vi "Set Color Table.vi"(10 "Color Table":T1={"Occupied Color"={"Value"=0, "Color"=0}, "Free Color"={"Value"=205, "Color"=16777215}, "Unknown Color"={"Value"=254, "Color"=13421772}}, 11 "Map Model in":refnum<class "Map Model.lvclass">) -> (3 "Map Model out":refnum<class "Map Model.lvclass">)   [LabVIEW 2020, in "Map Model.lvlib" / "Map Model.lvclass"]
uses:
  Map Model.lvclass
  Map Model.lvclass/Map Model.ctl
panel:
  # "NOTICE -- YOU MUST LEAVE THIS NOTICE IN PLACE.\n\nCopyright (c) 2017, LIANG LIU Shawn.Liu.cn@gmail.com\nAll rights reserved.\n\nRedistribution and use in source and binary forms, with or without modification, are permitted provided that the following conditions are met:\n-Redistributions of source code must retain the above copyright notice, this list of conditions and the following disclaimer.\n-Redistributions in binary form must reproduce the above copyright notice, this list of conditions and the following disclaimer in the documentation and/or other materials provided with the distribution.\n-Neither the name of the eLp nor the names of its contributors may be used to endorse or promote products derived from this software without specific prior written permission.\n\nTHIS SOFTWARE IS PROVIDED BY THE COPYRIGHT HOLDERS AND CONTRIBUTORS \"AS IS\" AND ANY EXPRESS OR IMPLIED WARRANTIES, INCLUDING, BUT NOT LIMITED TO, THE IMPLIED WARRANTIES OF MERCHANTABILITY AND FITNESS FOR A PARTICULAR PURPOSE ARE DISCLAIMED. IN NO EVENT SHALL THE COPYRIGHT HOLDER OR CONTRIBUTORS BE LIABLE FOR ANY DIRECT, INDIRECT, INCIDENTAL, SPECIAL, EXEMPLARY, OR CONSEQUENTIAL DAMAGES (INCLUDING, BUT NOT LIMITED TO, PROCUREMENT OF SUBSTITUTE GOODS OR SERVICES; LOSS OF USE, DATA, OR PROFITS; OR BUSINESS INTERRUPTION) HOWEVER CAUSED AND ON ANY THEORY OF LIABILITY, WHETHER IN CONTRACT, STRICT LIABILITY, OR TORT (INCLUDING NEGLIGENCE OR OTHERWISE) ARISING IN ANY WAY OUT OF THE USE OF THIS SOFTWARE, EVEN IF ADVISED OF THE POSSIBILITY OF SUCH DAMAGE."
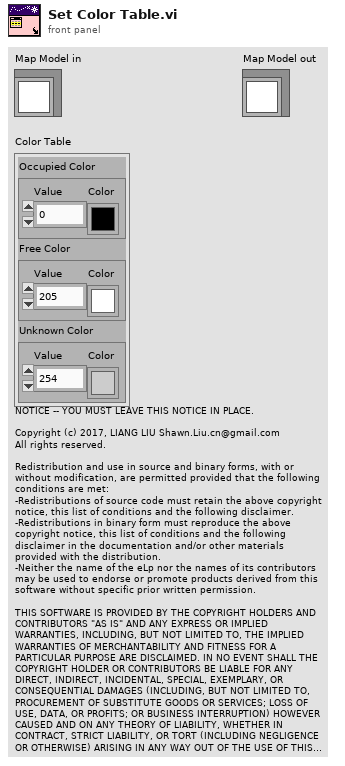
[diagram p1: front panel]
types:
  T1 = cluster{"Occupied Color":cluster{"Value":u8, "Color":u32}, "Free Color":cluster{"Value":u8, "Color":u32}, "Unknown Color":cluster{"Value":u8, "Color":u32}}
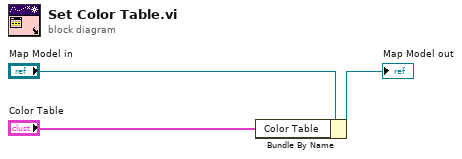
[diagram p0: block diagram]
diagram:
  n1 = Bundle By Name(cluster="Map Model in", "Color Table"="Color Table") -> (→"Map Model out":refnum<class "Map Model.lvclass">)
